vi "Get SMO Port.vi"(8 "error in (no error)":errorcluster, 11 "Inst.AH2500Instrument in":refnum<class "Inst.AH2500.lvclass">) -> (0 "error out":errorcluster, 2 "Port":u16, 3 "Inst.AH2500Instrument out":refnum<class "Inst.AH2500.lvclass">)   [LabVIEW 2019, in "Inst.AH2500.lvclass"]
uses:
  Inst.AH2500.lvclass
  <userlib>/LevyLab/Instrument Framework/Instrument Types/VSource/Instrument.VSource.lvclass
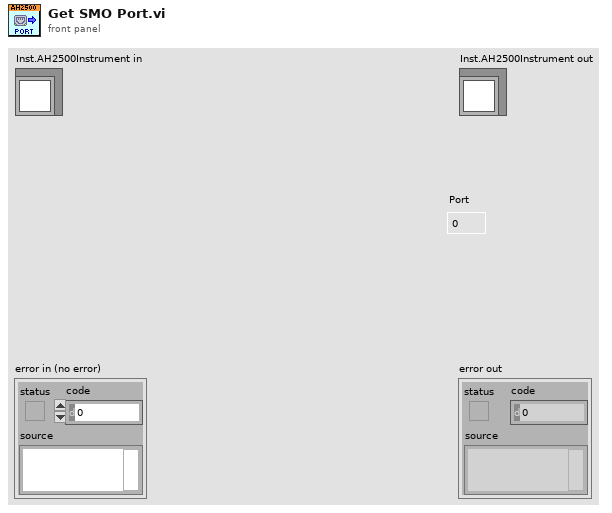
[diagram p1: front panel]
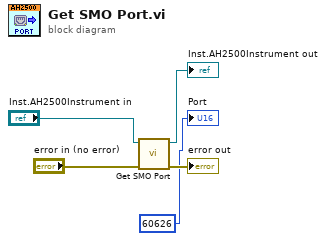
[diagram p0: block diagram]
diagram:
  n1 = call-parent "Get SMO Port.vi"("error in (no error)"="error in (no error)", "Instrument in"="Inst.AH2500Instrument in") -> ("error out"=→"error out":errorcluster, "Instrument out"=→"Inst.AH2500Instrument out":refnum<class "Inst.AH2500.lvclass">)  [unwired: 7 in, 1 out]
  "Port" <- u16 60626 ("Port")
